vi "Wait_untill_stopped_Peregrine.vi"(7 "Address":u8, 8 "error":errorcluster, 9 "stop":bool, 10 "milliseconds to wait":u32=200, 11 "Handle in":refnum<visa-resource-name>) -> (0 "error out":errorcluster, 1 "Emg stop":bool, 2 "Running":bool, 3 "Handle out":refnum<visa-resource-name>, 4 "Flags":T1, 6 "x .or. y?":bool)   [LabVIEW 2019]
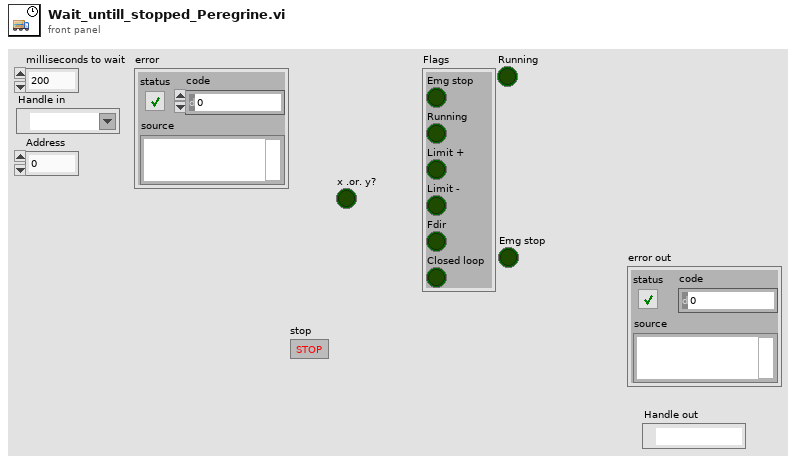
[diagram p1: front panel]
types:
  T1 = cluster{"Emg stop":bool, "Running":bool, "Limit +":bool, "Limit -":bool, "Fdir":bool, "Closed loop":bool}
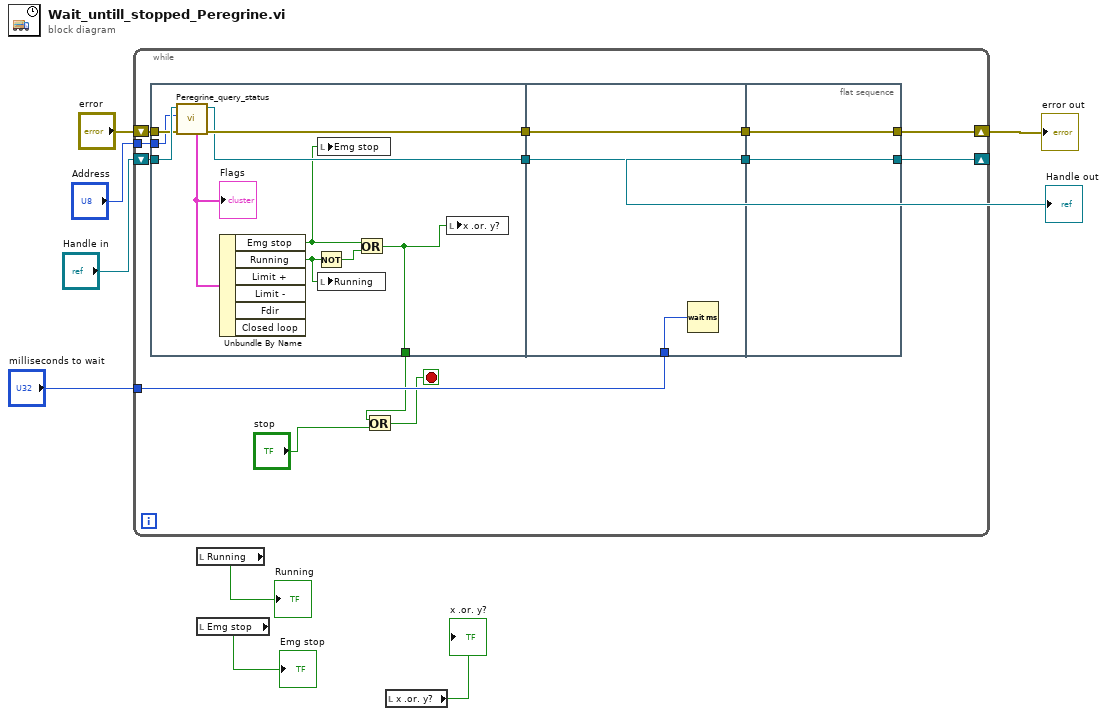
[diagram p0: block diagram]
diagram:
  n1 = while {
    tunnel: "milliseconds to wait" -> [w22]
    tunnel: "Address" -> [w19]
    shift-right: [w14] -> w5
    shift-left: "error" -> [w20]
    shift-right: [w13] -> w4
    shift-left: "Handle in" -> [w21]
    stop <- w10 stop-if-true
    n2 = flat-sequence {
      tunnel: w21 -> [w32]
      tunnel: w20 -> [w31]
      tunnel: w19 -> [w30]
      tunnel: [w29] -> w18
      tunnel: [w28] -> w16
      tunnel: [w23] -> w12
      tunnel: w22 -> [w35]
      tunnel: w18 -> [w34]
      tunnel: [w34] -> w17
      tunnel: w16 -> [w33]
      tunnel: [w33] -> w15
      tunnel: w17 -> [w37]
      tunnel: [w37] -> w14
      tunnel: w15 -> [w36]
      tunnel: [w36] -> w13
      frame #0 {
        n3 = call "Peregrine_query_status.vi"("error"=w31, "Address"=w30, "Handle in"=w32) -> ("error out"=w29:errorcluster, "Handle out"=w28:refnum<visa-resource-name>, "Flags"=w27:T1)  [unwired: 4 in, 2 out]
        "Flags" <- w27
        n4 = Unbundle By Name(w27) -> ("Emg stop"=w25:bool, "Running"=w24:bool)  [unwired: 4 out]
        n5 = Not(x=w24) -> (.not. x?=w26:bool)
        n6 = local write "Emg stop"(w25) -> ()
        n7 = local write "Running"(w24) -> ()
        n8 = Or(x=w25, y=w26) -> (x .or. y?=w23:bool)
        n9 = local write "x .or. y?"(w23) -> ()
      }
      frame #1 {
        n10 = Wait (ms)(milliseconds to wait=w35) -> ()  [unwired: 1 out]
      }
      frame #2 {
      }
    }
    n11 = Or(x=w12, y="stop") -> (x .or. y?=w10:bool)
  }
  "Handle out" <- w4
  "error out" <- w5
  n12 = local read "Running"() -> (→"Running":bool)
  n13 = local read "Emg stop"() -> (→"Emg stop":bool)
  n14 = local read "x .or. y?"() -> (→"x .or. y?":bool)
